vi "Catapult Set.vi"(9 "Catapult Configuration":T1, 10 "DevRef":string, 11 "SolenoidDevRef":T3={"DevStatus"={"status"=FALSE, "code"=0, "source"=""}, "Pneumatics Control Module"=0, "Forward Solenoid Channel"=enum."Invalid", "Reverse Solenoid Channel"=enum."Invalid"}) -> (3 "CatapultDevRefOut":T2={"Catapult State Reference"=refnum, "SolenoidDevRef"={"DevStatus"={"status"=FALSE, "code"=0, "source"=""}, "Pneumatics Control Module"=0, "Forward Solenoid Channel"=enum."Invalid", "Reverse Solenoid Channel"=enum."Invalid"}, "Catapult Configuration Reference"=refnum})   [LabVIEW 2015]
uses:
  <vilib>/Rock Robotics/WPI/Solenoid/WPI_SolenoidDevRef.ctl
  <vilib>/Rock Robotics/WPI/Solenoid/WPI_SolenoidChannel.ctl
  <userlib>/836 Library/Pneumatics/Catapult/836_CatapultDevRef.ctl
  <userlib>/836 Library/Pneumatics/Catapult/Catapult State.ctl
  <userlib>/836 Library/Pneumatics/Catapult/CatapultStateMachine.ctl
  <userlib>/836 Library/Pneumatics/Catapult/836_CatapultActions.ctl
  <userlib>/836 Library/Pneumatics/Catapult/Catapult Configuration.ctl
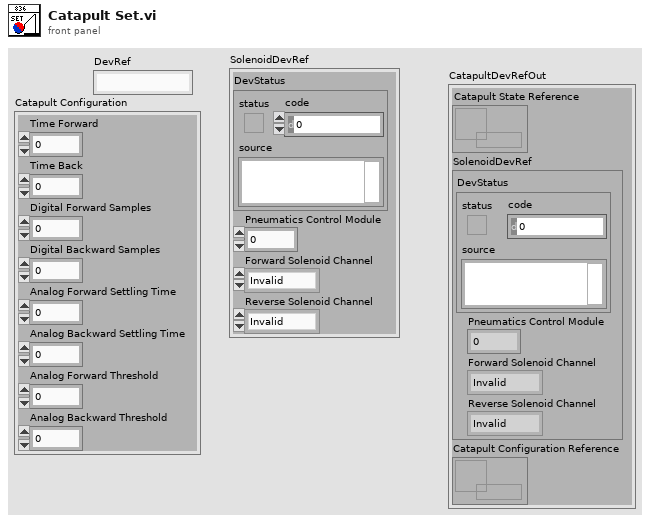
[diagram p1: front panel]
types:
  T1 = typedef "Catapult Configuration.ctl" = cluster{"Time Forward":u32, "Time Back":u32, "Digital Forward Samples":u32, "Digital Backward Samples":u32, "Analog Forward Settling Time":u32, "Analog Backward Settling Time":u32, "Analog Forward Threshold":sgl, "Analog Backward Threshold":sgl}
  T2 = typedef "836_CatapultDevRef.ctl" = cluster{"Catapult State Reference":refnum<data-value>, "SolenoidDevRef":T3, "Catapult Configuration Reference":refnum<data-value>}
  T3 = typedef "WPI_SolenoidDevRef.ctl" = cluster{"DevStatus":errorcluster, "Pneumatics Control Module":u8, "Forward Solenoid Channel":T4, "Reverse Solenoid Channel":T4}
  T4 = typedef "WPI_SolenoidChannel.ctl" = enum8{"Solenoid 0", "Solenoid 1", "Solenoid 2", "Solenoid 3", "Solenoid 4", "Solenoid 5", "Solenoid 6", "Solenoid 7", "Invalid"}
  T5 = typedef "Catapult State.ctl" = cluster{"Position":bool, "Initialize":bool, "First Action?":bool, "Current State":T6, "Multiuse Timer":u32, "Second Action":T7}
  T6 = typedef "CatapultStateMachine.ctl" = enum8{"Status", "Forward", "Back", "Timed Forward", "Timed Back", "Analog Forwad", "Analog Back", "Digital Forward", "Digital Back", "Off"}
  T7 = typedef "836_CatapultActions.ctl" = enum8{"Fire", "Fire Timed", "Fire Analog", "Fire Digital", "Retract", "Retract Timed", "Retract Analog", "Retract Digital", "Hold", "Toggle", "Toggle Timed", "Toggle Analog", "Toggle Digital"}
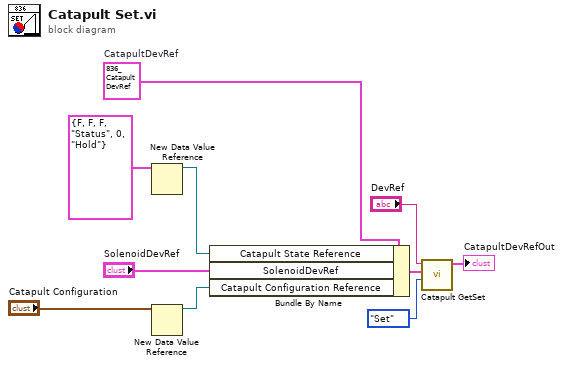
[diagram p0: block diagram]
diagram:
  w6 = T2 {"Catapult State Reference"=refnum, "SolenoidDevRef"={"DevStatus"={"status"=FALSE, "code"=0, "source"=""}, "Pneumatics Control Module"=0, "Forward Solenoid Channel"=enum."Invalid", "Reverse Solenoid Channel"=enum."Invalid"}, "Catapult Configuration Reference"=refnum}  # CatapultDevRef
  n1 = New Data Value Reference(data value=T5 {"Position"=FALSE, "Initialize"=FALSE, "First Action?"=FALSE, "Current State"=enum."Status", "Multiuse Timer"=0, "Second Action"=enum."Hold"} ("Cluster")) -> (data value reference=w4:refnum<data-value>)  [unwired: 1 in, 1 out]
  n2 = New Data Value Reference(data value="Catapult Configuration") -> (data value reference=w1:refnum<data-value>)  [unwired: 1 in, 1 out]
  n3 = Bundle By Name(cluster=w6, "Catapult State Reference"=w4, "SolenoidDevRef"="SolenoidDevRef", "Catapult Configuration Reference"=w1) -> (w8:T2)
  n4 = call <userlib>:"Catapult GetSet.vi"("Enum"=enum16{"Set", "Get"}."Set", "CatapultDevRef in"=w8, "DevRef"="DevRef") -> ("CatapulDevRef out"=→"CatapultDevRefOut":T2)  [unwired: 7 in, 1 out]
